vi "Get Operator Joystick State.vi"(8 "error in (no error)":errorcluster, 10 "Joystick State":T1, 11 "Operator in":refnum<class "Operator.lvclass">) -> (0 "error out":errorcluster, 3 "Operator out":refnum<class "Operator.lvclass">)   [LabVIEW 2014, in "Operator.lvlib" / "Operator.lvclass"]
uses:
  Operator.lvclass
  Joystick/Joystick Class/Joystick State.ctl
  Joystick/Joystick Class/Button State.ctl
  Joystick/Joystick Class/Axis State.ctl
  Joystick/Joystick Class/Joystick.lvclass
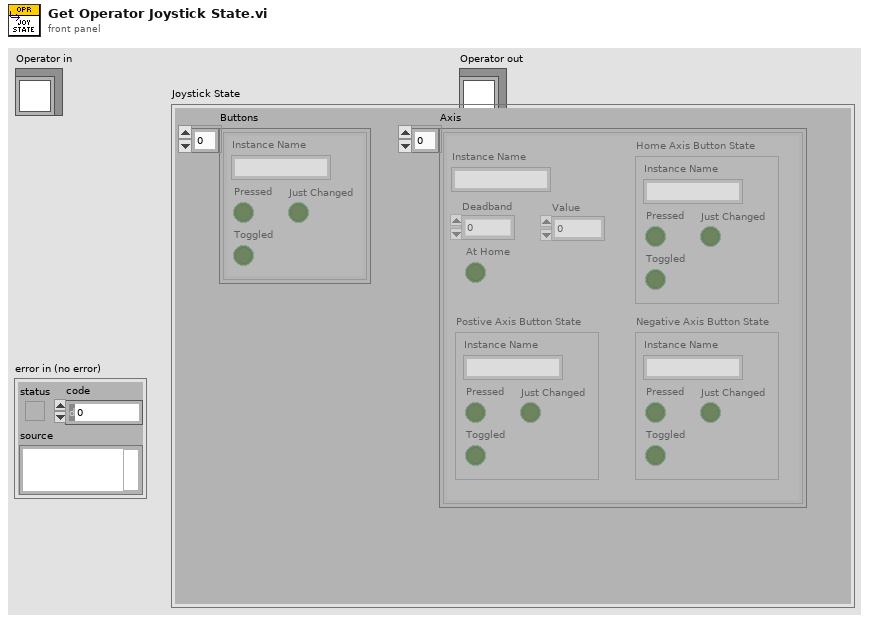
[diagram p1: front panel]
types:
  T1 = typedef "Joystick.lvlib/Joystick.lvclass/Joystick State.ctl" = cluster{"Buttons":T2[], "Axis":T3[]}
  T2 = typedef "Joystick.lvlib/Joystick.lvclass/Button State.ctl" = cluster{"Pressed":bool, "Instance Name":string, "Toggled":bool, "Just Changed":bool}
  T3 = typedef "Joystick.lvlib/Joystick.lvclass/Axis State.ctl" = cluster{"Instance Name":string, "Deadband":dbl, "Value":dbl, "At Home":bool, "Postive Axis Button State":T2, "Negative Axis Button State":T2, "Home Axis Button State":T2}
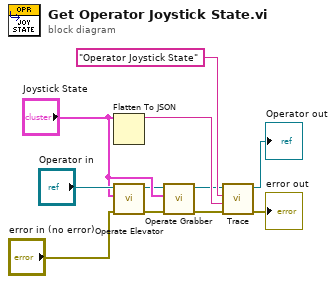
[diagram p0: block diagram]
diagram:
  n1 = Flatten To JSON(anything="Joystick State") -> (JSON string=w8:string)  [unwired: 2 in, 1 out]
  n2 = call-dynamic "Operate Elevator.vi"("error in (no error)"="error in (no error)", "Joystick State"="Joystick State", "Operator in"="Operator in") -> ("error out"=w3:errorcluster, "Operator out"=w6:refnum<class "Operator.lvclass">)  [unwired: 7 in]
  n3 = call-dynamic "Operate Grabber.vi"("error in (no error)"=w3, "Joystick State"="Joystick State", "Operator in"=w6) -> ("error out"=w2:errorcluster, "Operator out"=w5:refnum<class "Operator.lvclass">)  [unwired: 7 in]
  n4 = call-dynamic "Trace.vi"("error in (no error)"=w2, "System Message"=w8, "System Action"="Operator Joystick State", "System Actor in"=w5) -> ("error out"=→"error out":errorcluster, "System Actor out"=→"Operator out":refnum<class "Operator.lvclass">)  [unwired: 6 in]
